vi "Show Detected Current Indicator.vi"(8 "error in":errorcluster, 11 "ProXR in":refnum<class "ProXR.lvclass">) -> (0 "error out":errorcluster, 3 "ProXR out":refnum<class "ProXR.lvclass">)   [LabVIEW 2019, in "ProXR.lvlib" / "ProXR.lvclass"]
uses:
  Library/ProXR.lvclass
  C:/Users/Public/Documents/Development/builds/Instruments/DIG_IO.lvlibp/Library/DIG_IO.lvclass
  builds/Instruments/DIG_IO.lvlibp/Accessors/Read Detected_Current_ref.vi
  builds/Instruments/DIG_IO.lvlibp/Accessors/Read Current_Query_ref.vi
  builds/Instruments/DIG_IO.lvlibp/Accessors/Write Detected_Current_ref.vi
  builds/Instruments/DIG_IO.lvlibp/Accessors/Write Current_Query_ref.vi
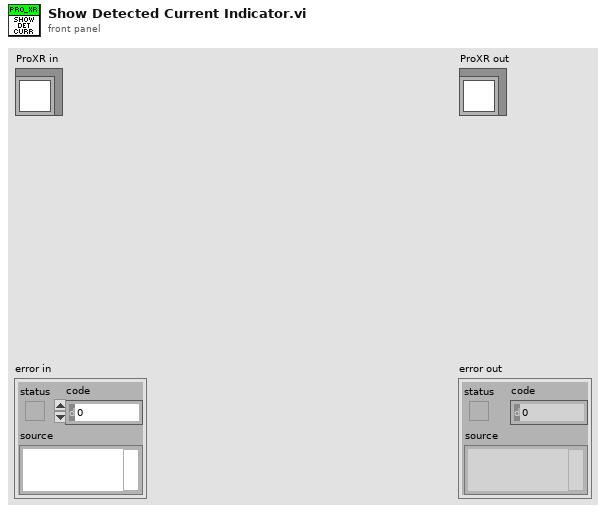
[diagram p1: front panel]
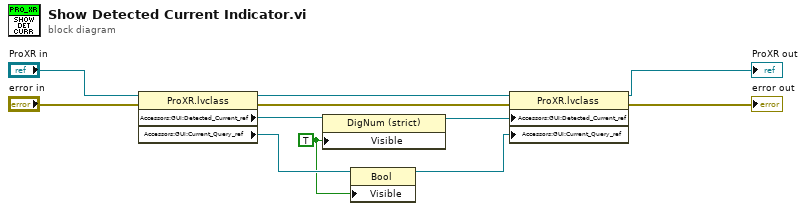
[diagram p0: block diagram]
diagram:
  w6 = TRUE ("Visible")
  n1 = property class="ProXR.lvclass"(reference="ProXR in", error in="error in") -> (reference out=w4:refnum<class "ProXR.lvclass">, error out=w9:errorcluster, "Accessors:GUI:Detected_Current_ref"=w8:refnum<vi>, "Accessors:GUI:Current_Query_ref"=w7:refnum<vi>)
  n2 = property class="DigNum (strict)"(reference=w8, "Visible"=w6) -> (reference out=w2:refnum<vi>)  [unwired: 1 in, 1 out]
  n3 = property class="Bool"(reference=w7, "Visible"=w6) -> (reference out=w1:refnum<vi>)  [unwired: 1 in, 1 out]
  n4 = property class="ProXR.lvclass"(reference=w4, error in=w9, "Accessors:GUI:Detected_Current_ref"=w2, "Accessors:GUI:Current_Query_ref"=w1) -> (reference out=→"ProXR out":refnum<class "ProXR.lvclass">, error out=→"error out":errorcluster)
